vi "RobotToMapCoOrd.vi"(8 "Robot Y":dbl, 11 "Robot X":dbl) -> (2 "RobotXandYonMap":cluster{"X":i32, "Y":i32})   [LabVIEW 2014]
panel:
  # "This VI converts robot true coordinates to Map Coordinates"
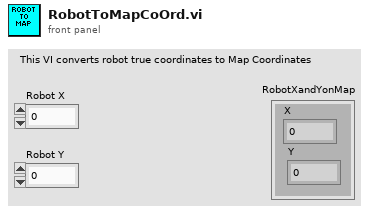
[diagram p1: front panel]
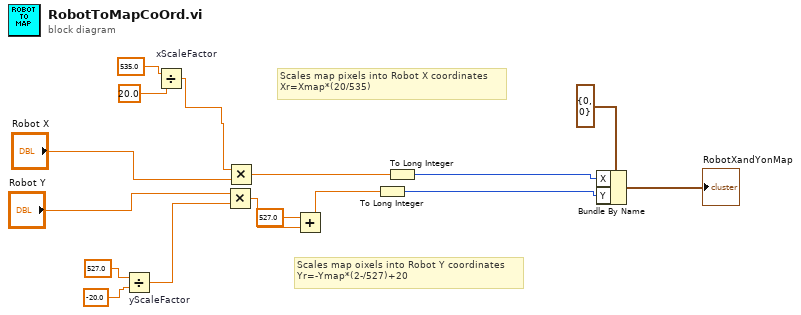
[diagram p0: block diagram]
diagram:
  # "Scales map oixels into Robot Y coordinates\nYr=-Ymap*(2-/527)+20"
  # "Scales map pixels into Robot X coordinates\nXr=Xmap*(20/535)"
  n1 = Divide "yScaleFactor"(x=527.0 ("y"), y=-20.0 ("x")) -> (x/y=w5:dbl)
  n2 = Divide "xScaleFactor"(x=535.0 ("y"), y=20.0 ("x")) -> (x/y=w8:dbl)
  n3 = Multiply(x="Robot Y", y=w5) -> (x*y=w12:dbl)
  n4 = Multiply(x=w8, y="Robot X") -> (x*y=w11:dbl)
  n5 = Add(x=527.0, y=w12) -> (x+y=w13:dbl)
  n6 = To Long Integer(number=w13) -> (32bit integer=w9:i32)
  n7 = To Long Integer(number=w11) -> (32bit integer=w10:i32)
  n8 = Bundle By Name "Bundle By Name"(cluster=cluster{"X":i32, "Y":i32} {"X"=0, "Y"=0} ("RobotXandY"), "X"=w10, "Y"=w9) -> (→"RobotXandYonMap":cluster{"X":i32, "Y":i32})
